vi "data handle.vi"(0 "unit":u16(ring) items=["s"=0, "ms"=3, "us"=6, "ns"=9], 1 "Y":dbl[](array[numeric]), 2 "X Increment (input)":dbl, 3 "InitialX (input)":dbl) -> (7 "T":dbl[](array[numeric]), 8 "T Y":dbl[][](array[numeric]), 9 "X Increment(by unit)":dbl, 10 "Initial X(by unit)":dbl caption="Initial X" format="%^.3e")   [LabVIEW 2018]
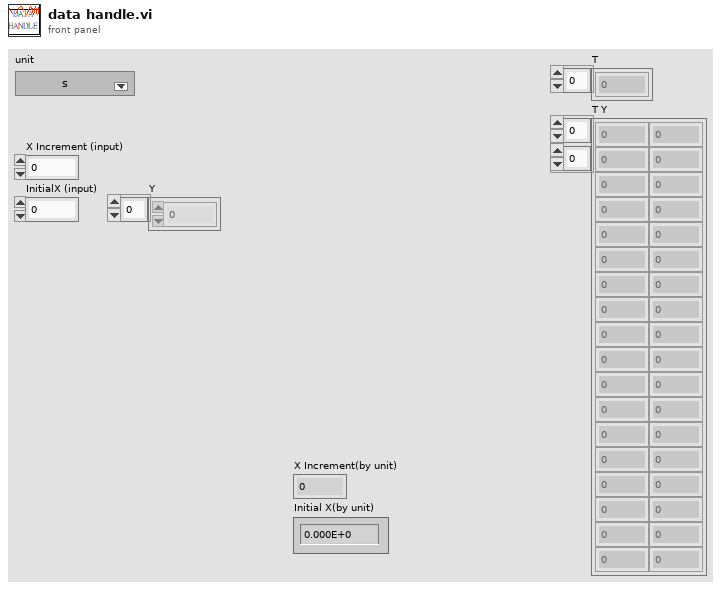
[diagram p1: front panel]
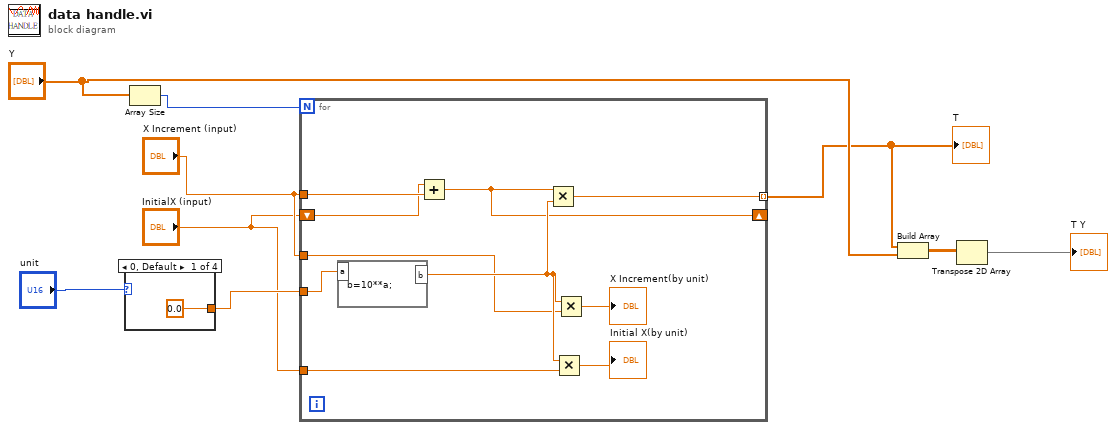
[diagram p0: block diagram]
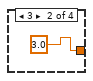
[diagram p2: hidden frame]
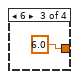
[diagram p3: hidden frame]
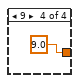
[diagram p4: hidden frame]
diagram:
  n1 = case shown="0, Default" "unit" {
    tunnel: [0.0 3.0 6.0 9.0] -> w9
    frame 0, Default {
    }
    frame 3 {
    }
    frame 6 {
    }
    frame 9 {
    }
  }
  n2 = Array Size(array="Y") -> (size(s)=w7:i32)
  n3 = for {
    N: w7 -> [_]
    tunnel: [w23] -> w3 mode=indexing
    shift-right: [w15] -> _
    shift-left: "InitialX (input)" -> [w14]
    tunnel: w9 -> [w22]
    tunnel: "X Increment (input)" -> [w19]
    tunnel: "InitialX (input)" -> [w17]
    tunnel: "X Increment (input)" -> [w16]
    n4 = formula code="b=10**a;"("a"=w22) -> ("b"=w18:dbl)
    n5 = Add(x=w14, y=w19) -> (x+y=w15:dbl)
    n6 = Multiply(x=w15, y=w18) -> (x*y=w23:dbl)
    n7 = Multiply(x=w18, y=w17) -> (x*y=→"Initial X(by unit)":dbl)
    n8 = Multiply(x=w18, y=w16) -> (x*y=→"X Increment(by unit)":dbl)
  }
  "T" <- w3
  n9 = Build Array(w3, "Y") -> (w6:dbl[][])
  n10 = Transpose 2D Array(2D array=w6) -> (transposed array=→"T Y":dbl[][])
